vi "proj.versao2.vi"() -> ()   [LabVIEW 2025]
uses:
  <vilib>/Utility/file.llb/Read Delimited Spreadsheet (DBL).vi
  <vilib>/Utility/file.llb/Read Delimited Spreadsheet (string).vi
panel:
  in  "Tab Control":enum32{"Manual", "Processamento", "Recuperação"}(tab)
  out "O programa":string="O programa foi desenvolvido com o objetivo de visualizar a analisar dados fisiológicos de um paciente durante a realização de exercício físico leve, como caminhada. A aplicação realiza a leitura de um arquivo contendo as medições registradas pelo dispisitivo de monitoramento e apresenta, de forma gráfica, os pricipais parâmetros coletados: SpO2, BPM e PAI(%). \n\nPor meio da interface do programa, é possível acompanhar o comportamento dessas variáveis ao longo do tempo, bem como identificar os valores máximos e mínimos registrados durante o teste. Além disso, o sistema permite a análise do período de recuperação do paciente após o exercício, possibilitando avaliar o tempo necessário para que os parâmetros fisiológicos retornem a níveis próximos aos de repouso. Dessa forma, o programa auxilia na interpretação dos dados coletados e na avaliação da resposta fisiológica do paciente ao exercício."
  out "Recuperação":string="Na aba Recuperação, são analisadas as medidas de SpO2 registradas no momento em que o paciente se encontra em repouso, após a realização da caminhada. O objetivo dessa etapa é avaliar o tempo necessário para que o paciente retorne aos seus valores fisiológicos de repouso, indicando o processo de restabelecimento após o exercício. Como o tempo de caminhada e de recuperação pode variar entre os pacientes, a definição desses intervalos deve ser ajustada manualmente no gráfico, de acordo com o período correspondente a cada fase do teste.\n\nO primeiro gráfico deve representar toda a jornada do paciente, desde o momento em que o dispositivo de medição é colocado até o final do teste. Já o segundo gráfico deve apresentar apenas o período de recuperação, ou seja, o intervalo correspondente ao momento em que o paciente está parado após a caminhada.  Como o tempo de caminhada e de recuperação pode variar entre os pacientes, a definição desses intervalos deve ser ajustada manualmente no gráfico, de acordo com cada teste realizado."
  out "Processamento":string="Na aba Processamento, são apresentados três gráficos correspondentes às variáveis monitoradas durante o exercício: SpO2 (%), BPM e PAI (%), respectivamente. Cada gráfico exibe o comportamento dessas variáveis ao longo do tempo, sendo o tempo representado em segundos no eixo horizontal. Ao lado de cada gráfico, são exibidos os valores máximo e mínimo registrados para a respectiva variável, permitindo uma visualização rápida das variações ocorridas durante o período analisado."
  in  "insira o arquivo":path
  out "Waveform Graph (spo2)":dbl[](graph)
  out "max value 3":dbl
  out "min value 3":dbl
  out "Waveform Graph 2 (BPM)":dbl[](graph)
  out "Waveform Graph (PAI) 2":dbl[](graph)
  out "max value":dbl
  out "min value":dbl
  out "max value 2":dbl
  out "min value 2":dbl
  out "Waveform Graph (spo2) 3":dbl[](graph)
  out "Waveform Graph (sp02) 2":dbl[](graph)
  out "first row":string[](array[string])
  out "all rows":dbl[][](array[numeric]) format="%_4g"
  # "em andamento: \n\n1) resolver o float que não aparece. \nsugestão: multiplicar tudo por 100\najustar o excel por células e não por vírgulas\nfazer de outra forma\n\n2) graficar\n\nColocar parâmetro PAI no gráfico mesmo sem casa decimal. \n\nE depois colocar valores de maximo e minimo em um visor do lado. prra isso pesquise\ntodas as funçoes array"
  # "manual: colocar dúvidas que forem aparecendo a medida que os usuários forem usando. pensar em uma caixinha de perguntas que permita\nao usuário deixar dúvidas sobre o programa\n\nprocessamento: gráficos principais\n\nrecuperação: pegaremos as medidas no momento em que os pacientes estiverem parados se recuperando da caminhada.\no tempo de caminhada muda de acordo com o paciente, essa mudança de intervalos deve ser feita manualmente"
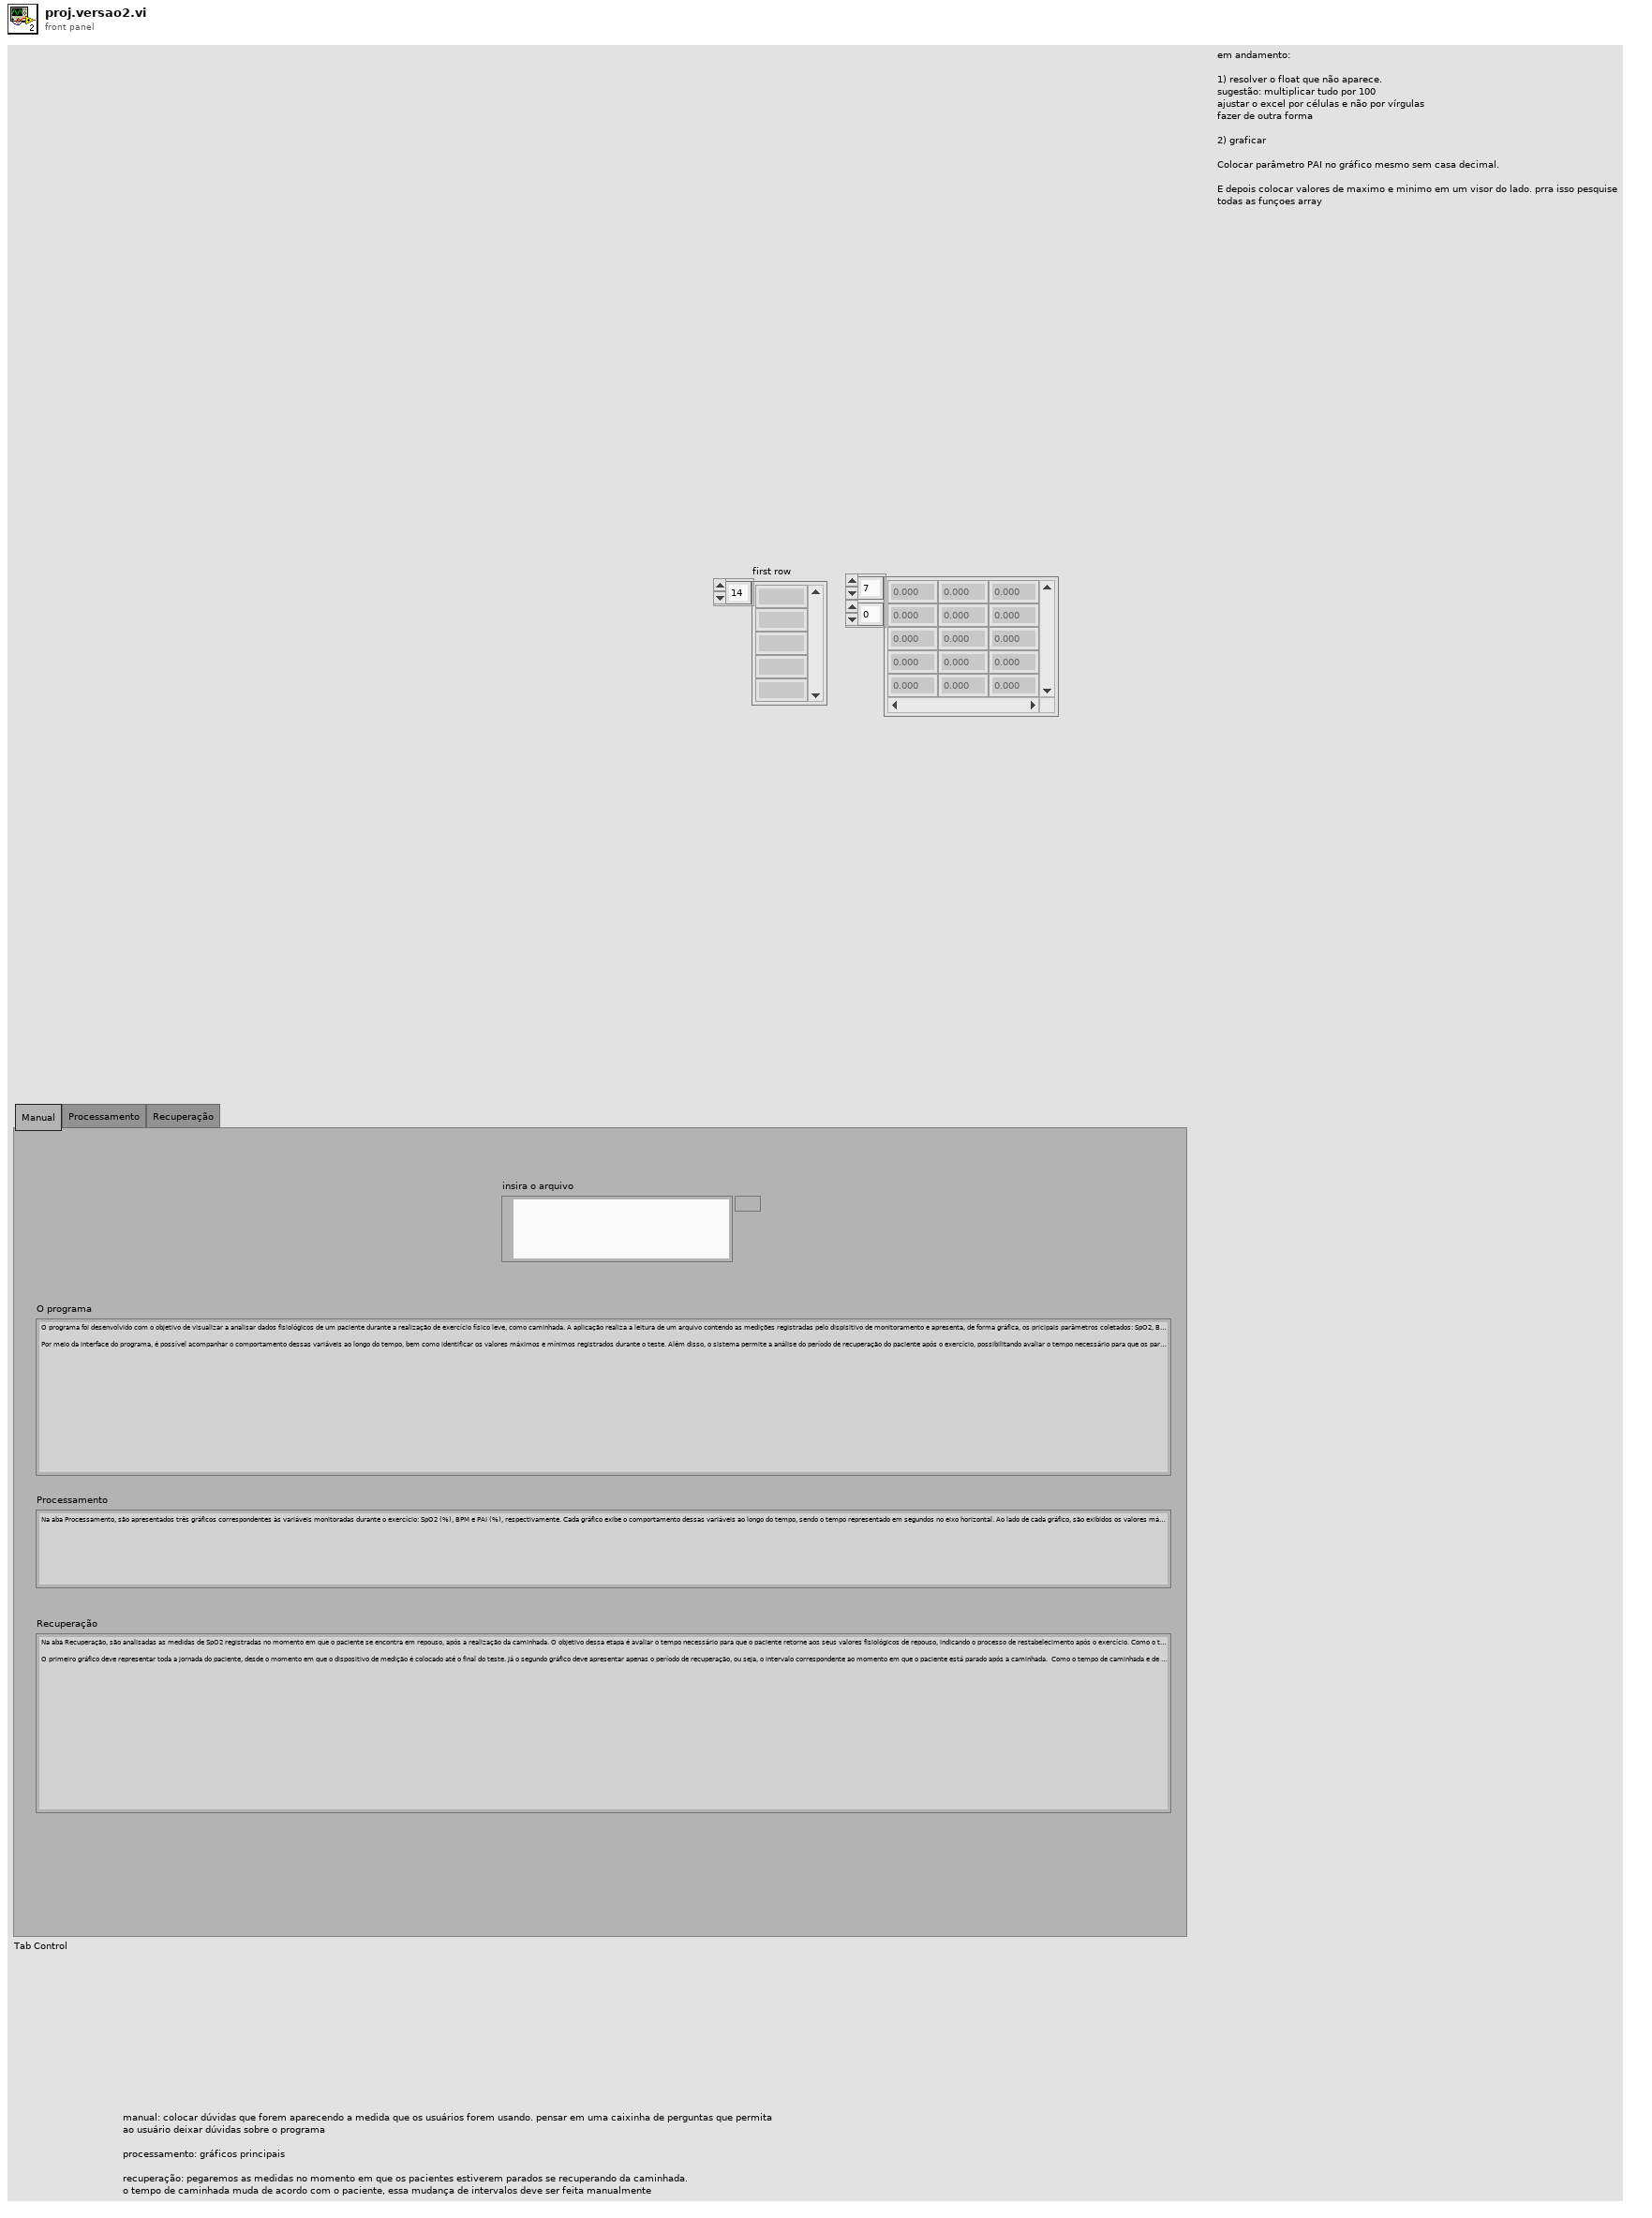
[diagram p1: front panel]
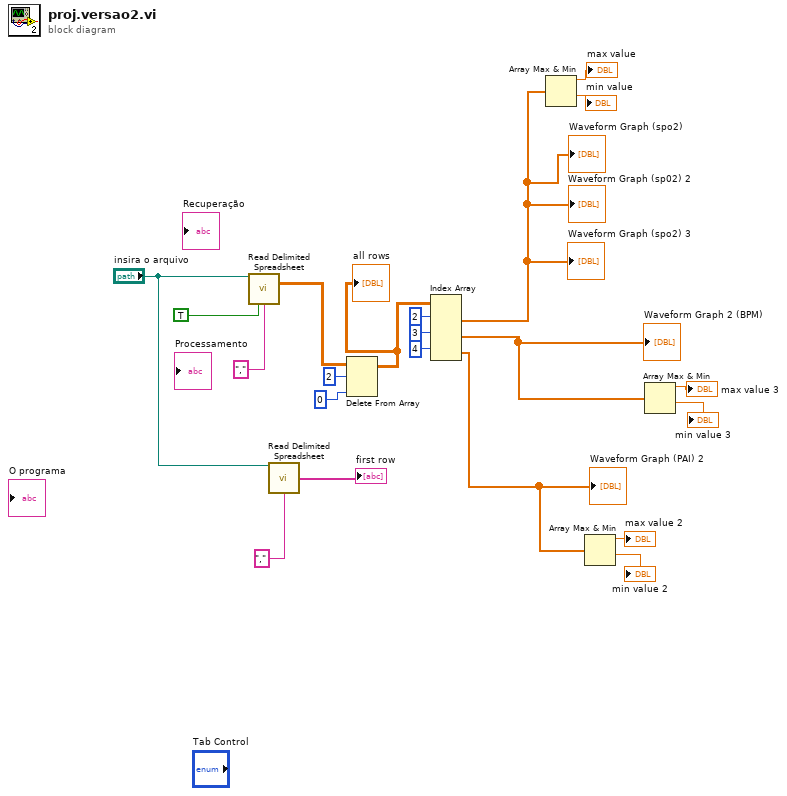
[diagram p0: block diagram]
diagram:
  n1 = call-poly <vilib>:"Read Delimited Spreadsheet.vi"("file path (dialog if empty)"="insira o arquivo", "transpose? (F)"=TRUE, "delimiter (\\t)"="," ("delimiter (\\t)")) -> ("all rows"=w15:dbl[][])  [unwired: 7 in, 5 out]
  n2 = call-poly <vilib>:"Read Delimited Spreadsheet.vi"("file path (dialog if empty)"="insira o arquivo", "delimiter (\\t)"="," ("delimiter (\\t)")) -> ("first row"=→"first row":string[])  [unwired: 8 in, 5 out]
  n3 = Delete From Array(array=w15, length=2, index (col)=0 ("disabled index (col)")) -> (array with subset deleted=w13:dbl[][])  [unwired: 1 in, 1 out]
  "all rows" <- w13
  n4 = Index Array(array=w13, index (row) #1=2 ("index (row)"), index (row) #2=3 ("index (row)"), index (row) #3=4 ("index (row)")) -> (element #1=w1:dbl[], element #2=w4:dbl[], element #3=w7:dbl[])  [unwired: 3 in]
  "Waveform Graph (spo2)" <- w1
  "Waveform Graph 2 (BPM)" <- w4
  "Waveform Graph (PAI) 2" <- w7
  "Waveform Graph (sp02) 2" <- w1
  "Waveform Graph (spo2) 3" <- w1
  n5 = Array Max & Min(array=w1) -> (max value=→"max value":dbl, min value=→"min value":dbl)  [unwired: 2 out]
  n6 = Array Max & Min(array=w7) -> (max value=→"max value 2":dbl, min value=→"min value 2":dbl)  [unwired: 2 out]
  n7 = Array Max & Min(array=w4) -> (max value=→"max value 3":dbl, min value=→"min value 3":dbl)  [unwired: 2 out]
